vi "KoordListGUI.vi"() -> ()   [LabVIEW 2011]
uses:
  <vilib>/Utility/error.llb/whitespace.ctl
panel:
  in  "Detector":u16(ring) items=["scan", "pike"]
  in  "Positions":i32=12
  in  "Registerkarte":T1(tab)=enum."Size"
  in  "Save":bool
  in  "Load":bool
  in  "slide-center [m]":cluster{"X":dbl, "Y":dbl}={"X"=0.0106, "Y"=0.004}
  in  "slide-size [m]":cluster{"X":dbl, "Y":dbl}={"X"=0.02, "Y"=0.01}
  in  "step":cluster{"Stepx":dbl, "Stepy":dbl}={"Stepx"=0.0006, "Stepy"=0.0006} {"Stepy" format="%#_6p"; "Stepx" format="%#_6p"}
  out "Objective X":dbl=10.0
  in  "ReadSize":bool
  out "y":i32=3
  out "x":i32=4
  in  "max":cluster{"maxX":dbl, "maxY":dbl}={"maxX"=0.011708333333333331, "maxY"=0.0028645833333333336} {"maxY" format="%#_6p"; "maxX" format="%#_6p"}
  in  "min":cluster{"MinX":dbl, "MinY":dbl}={"MinX"=0.0044166666666666625, "MinY"=-0.0031249999999999993} {"MinY" format="%#_6p"; "MinX" format="%#_6p"}
  out "Image":T2(plugin-control)
  in  "create list":bool
  out "Mouse position":cluster{"x":dbl, "y":dbl}={"x"=1.9429894176211716e-14, "y"=99.99999999999996} {"y" format="%#_6p"; "x" format="%#_6p"}
  in  "List":i32(listbox)=-1
  out "experimet":string="steve7"
  in  "Cancel":bool
  in  "Run":bool
  in  "State":T3(ring)=enum."close"
  out "Next is":i32
  out "Numerisch":dbl=0.00474167
  out "String":string="stage.y.set"
  out "stage notification":string=" 0.011600 ,0.0000"
  in  "End":bool
  # "Coordinates"
  # "Till-stage: 0.01248/0.01235\nPrior: 0,05703/0,03722\nAsi is 0.006/0"
  # "default size 0.050/0.025"
  # "of last image \ndone with this\ndetector"
  # "(Image center!)"
  # "Debug"
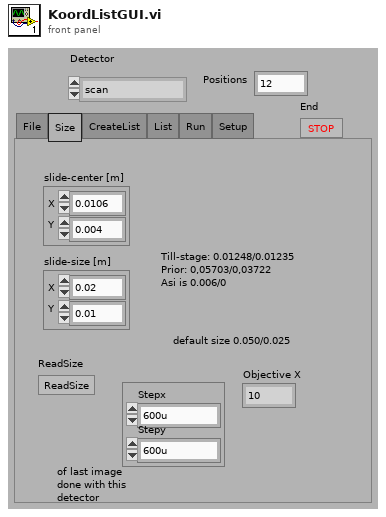
[diagram p1: front panel]
types:
  T1 = enum32{"File", "Size", "CreateList", "List", "Run", "Setup"}
  T2 = typedef "IMAQ Image.ctl" = refnum<image>
  T3 = enum16{"idle", "start", "move", "image", "stop", "close"}
  T4 = enum16{"None/#Datasets", "Clear", "TagValueOf#", "AddValues", "ReadValue", "ChangeValue", "Get all"}
  T5 = typedef "Image Type" = u32
  T6 = typedef "whitespace.ctl" = u16
  T7 = cluster{"Global Rectangle":i32[], "Contours":cluster{"Contour Type":u32, "ROI Type":u32, "Points":i32[]}[]}
  T8 = typedef "IMAQ Rectangle" = cluster{"Left":i32, "Top":i32, "Right":i32, "Bottom":i32, "Rotation":dbl}
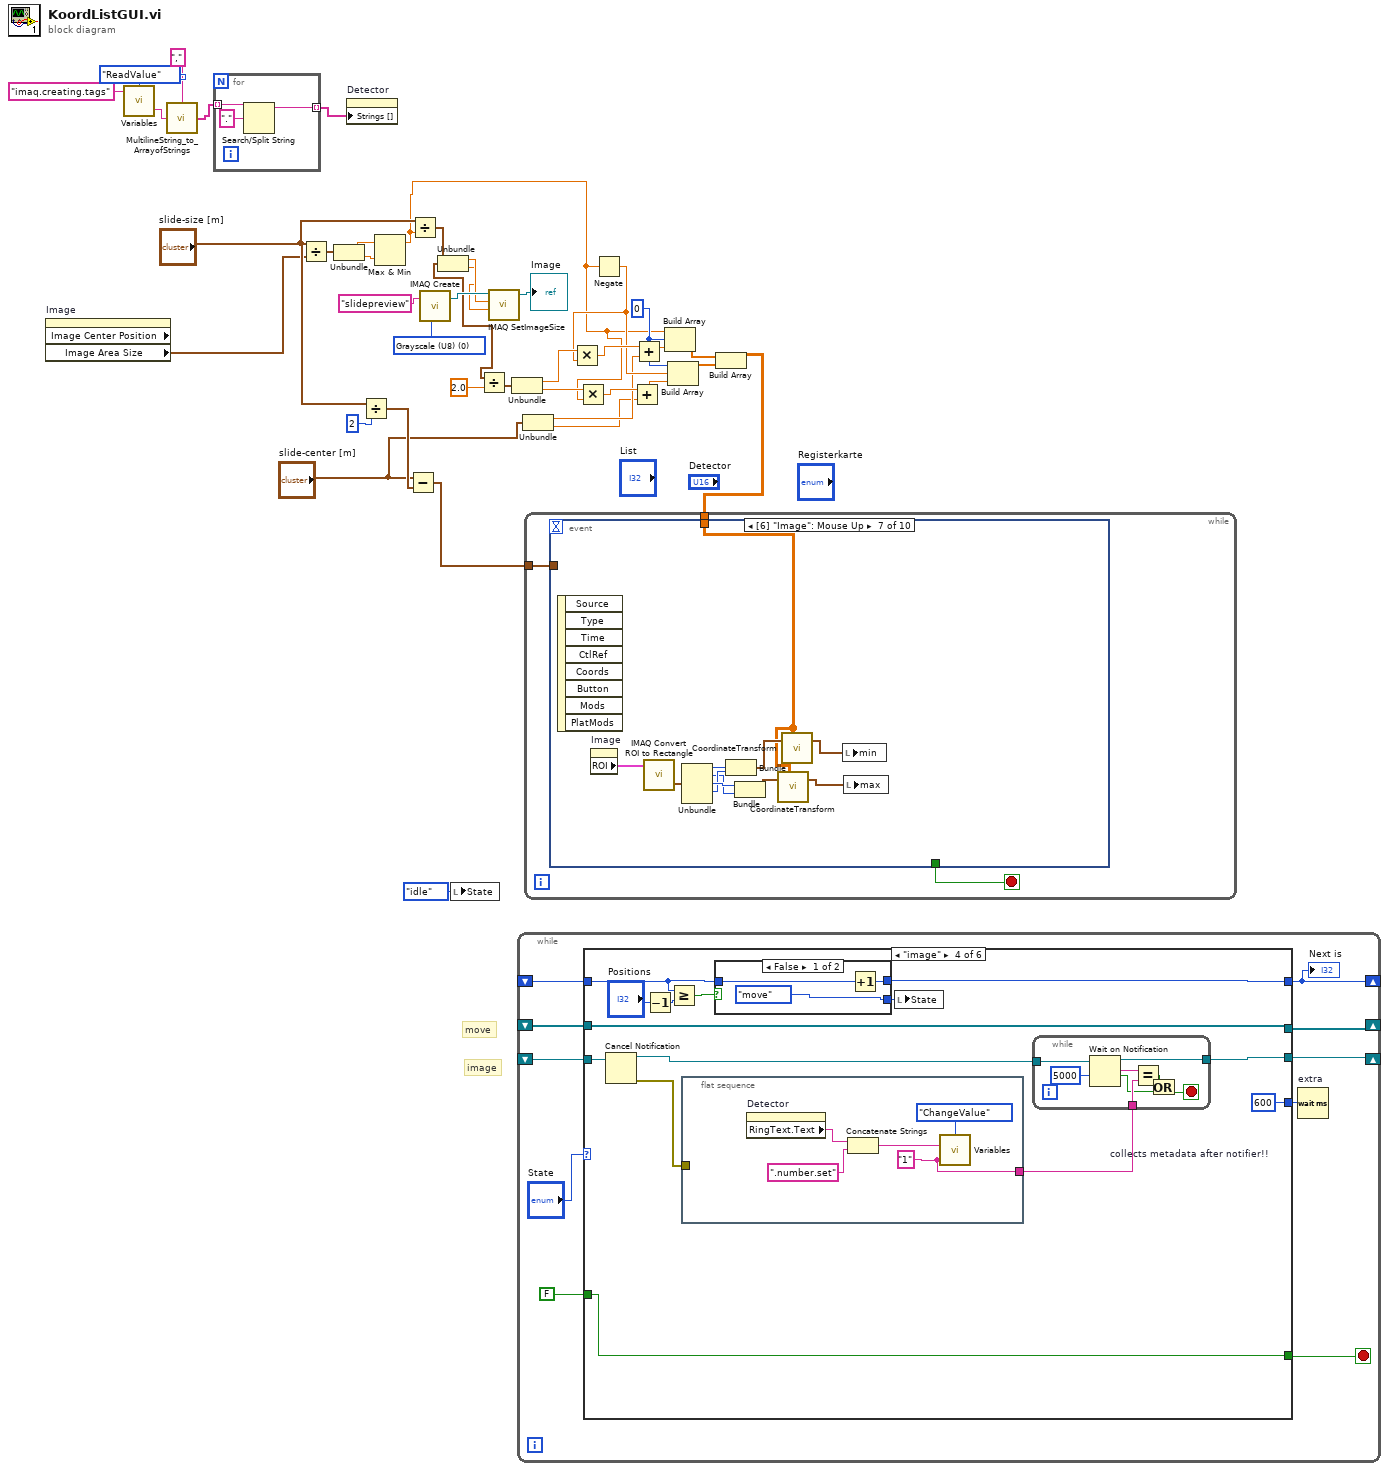
[diagram p0: block diagram]
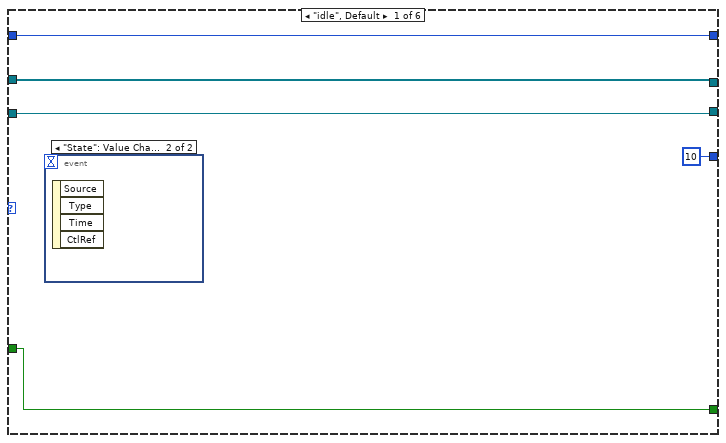
[diagram p2: hidden frame]
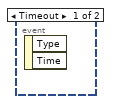
[diagram p3: hidden frame]
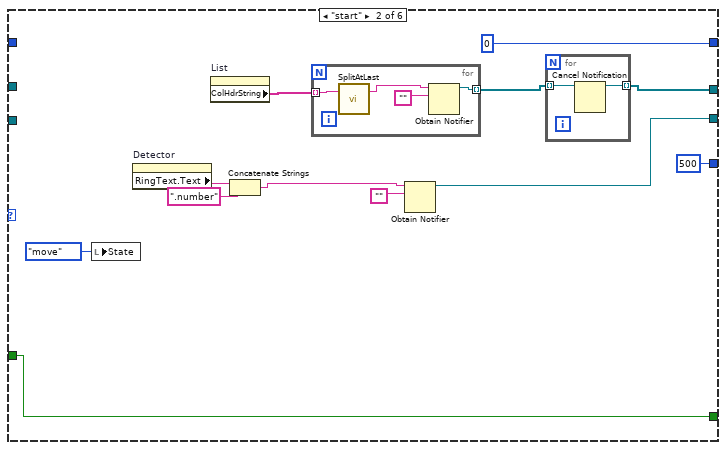
[diagram p4: hidden frame]
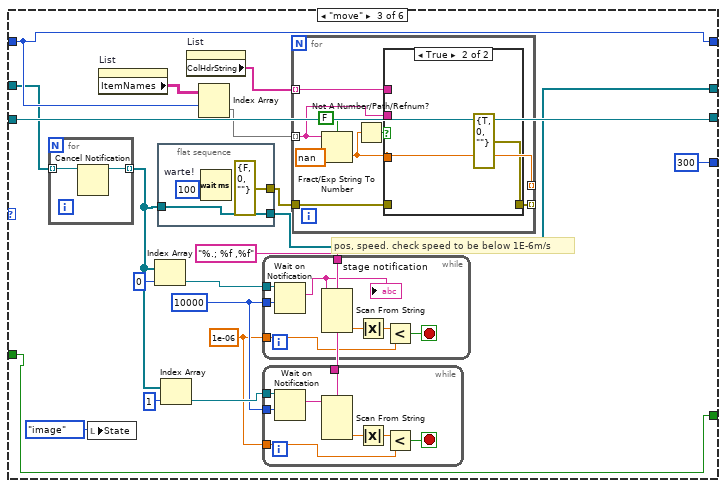
[diagram p5: hidden frame]
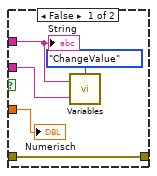
[diagram p6: hidden frame]
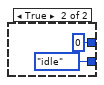
[diagram p7: hidden frame]
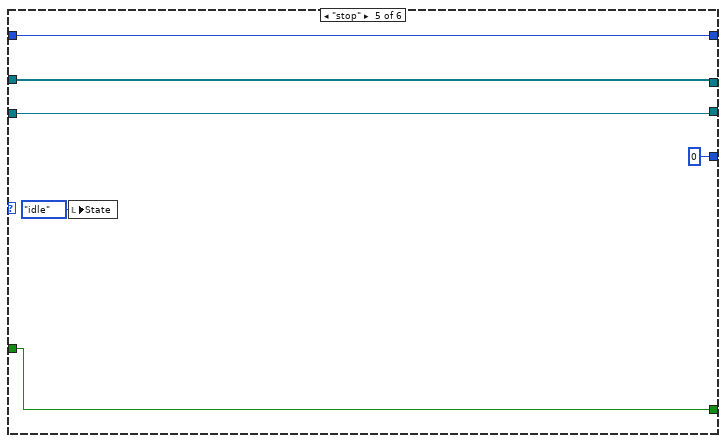
[diagram p8: hidden frame]
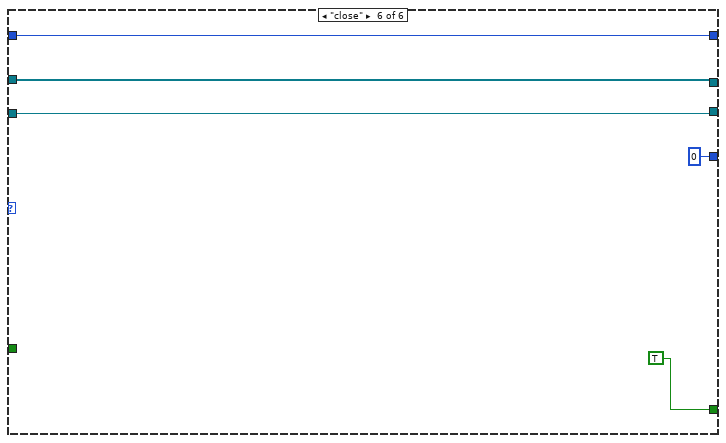
[diagram p9: hidden frame]
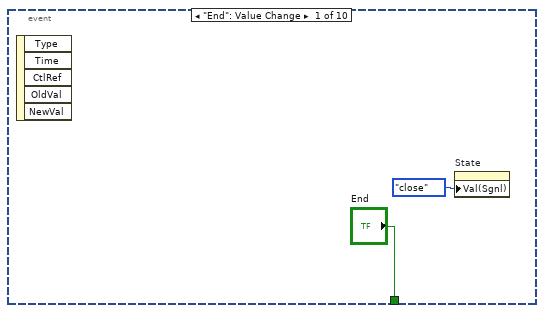
[diagram p10: hidden frame]
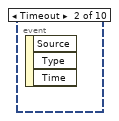
[diagram p11: hidden frame]
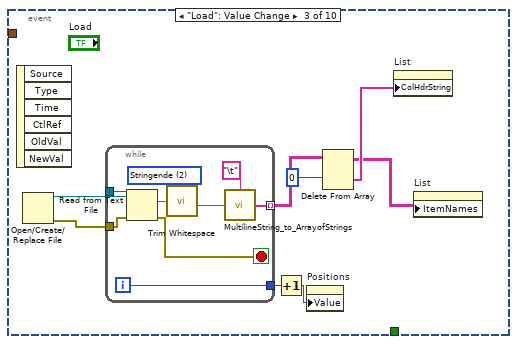
[diagram p12: hidden frame]
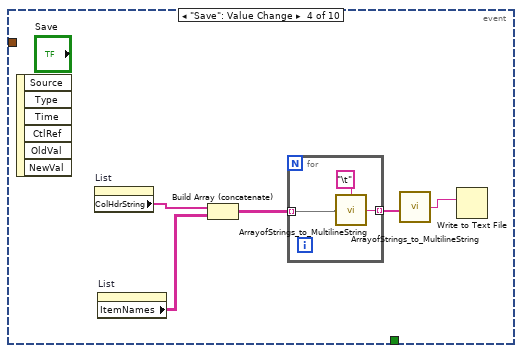
[diagram p13: hidden frame]
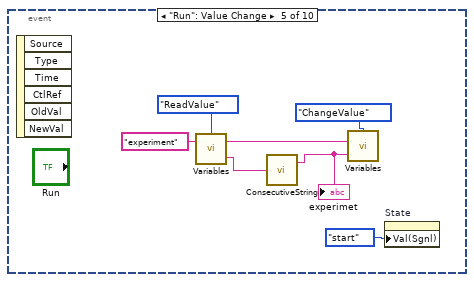
[diagram p14: hidden frame]
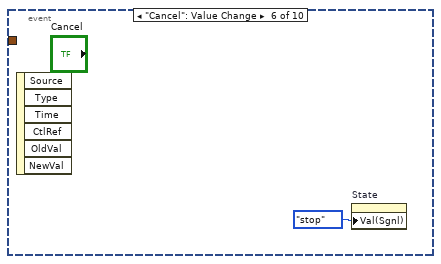
[diagram p15: hidden frame]
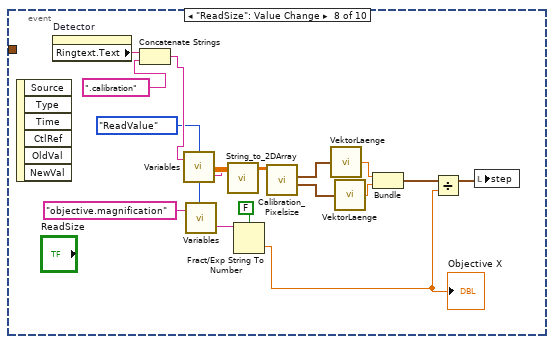
[diagram p16: hidden frame]
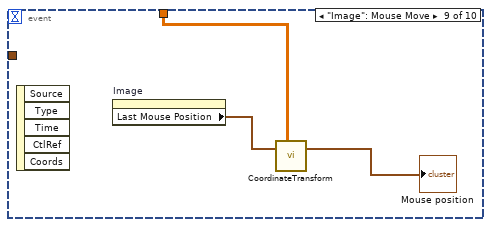
[diagram p17: hidden frame]
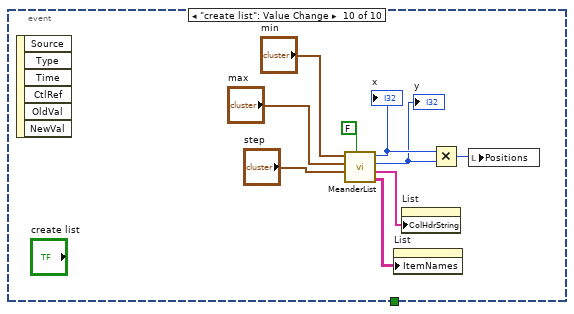
[diagram p18: hidden frame]
diagram:
  w23 = 0
  w38 = T5 0 items=["Grayscale (U8)", "Grayscale (I16)", "Grayscale (SGL)", "Complex (CSG)", "RGB (U32)", "HSL (U32)", "RGB (U64)"] ("Image Type")
  # "image"
  # "move"
  n1 = property on="Image" class="ImageControl" props=["Image Center Position", "Image Area Size"]() -> ("Image Area Size"=w21:cluster{"Width":u32, "Height":u32})  [unwired: 2 in, 3 out]
  n2 = call "Variables.vi"("Tag in"="imaq.creating.tags", "Command"=T4."ReadValue") -> ("value out"=w11:string)  [unwired: 1 in, 2 out]
  n3 = call "MultilineString_to_ArrayofStrings.vi"("String 1"=w11, "NewLineString"=",") -> ("String Array"=w9:string[])
  n4 = for {
    tunnel: w9 -> [w42] mode=indexing
    tunnel: [w41] -> w8 mode=indexing
    n5 = Search/Split String(string=w42, search string/char (-)=".") -> (substring before match=w41:string)  [unwired: 1 in, 2 out]
  }
  n6 = Divide(x="slide-size [m]", y=w21) -> (x/y=w34:cluster{dbl, dbl})
  n7 = Unbundle(w34) -> (w33:dbl, w32:dbl)
  n8 = property on="Detector" class="Ring (strict)"("Strings []"=w8) -> ()  [unwired: 2 in, 2 out]
  n9 = Divide(x="slide-size [m]", y=2) -> (x/y=w28:cluster{"X":dbl, "Y":dbl})
  n10 = Max & Min(x=w33, y=w32) -> (max(x,y)=w14:dbl)  [unwired: 1 out]
  n11 = Subtract(x="slide-center [m]", y=w28) -> (x-y=w27:cluster{"X":dbl, "Y":dbl})
  n12 = Divide(x="slide-size [m]", y=w14) -> (x/y=w18:cluster{"X":dbl, "Y":dbl})
  n13 = call "IMAQ Create"("Image Name"="slidepreview", "Image Type"=w38) -> ("New Image"=w37:T2)  [unwired: 2 in, 2 out]
  n14 = Unbundle(w18) -> ("X"=w36:dbl, "Y"=w35:dbl)
  n15 = local write "State"(T3."idle" ("State")) -> ()
  n16 = Divide(x=w18, y=2.0) -> (x/y=w17:cluster{"X":dbl, "Y":dbl})
  n17 = call "IMAQ SetImageSize"("Y Resolution"=w35, "X Resolution"=w36, "Image"=w37) -> ("Image Out"=→"Image":T2)  [unwired: 1 in, 2 out]
  n18 = Unbundle(w17) -> ("X"=w20:dbl, "Y"=w19:dbl)
  n19 = while {
    shift-right: [w51] -> _
    shift-left: _ -> [w52]
    shift-right: [w50] -> _
    shift-left: _ -> [w49]
    shift-right: [w44] -> _
    shift-left: _ -> [w48]
    stop <- w47 stop-if-true
    n20 = case shown="\"image\"" "State" {
      tunnel: w52 -> [w57 _ w82 w143 w166 w171]
      tunnel: [w57 w61 w81 w143 w166 w171] -> w51
      tunnel: [w56 w67 w94 w142 w165 w170] -> w50
      tunnel: w49 -> [w56 _ w94 w132 w165 w170]
      tunnel: w48 -> [w55 _ w89 w137 w167 w172]
      tunnel: [w55 0 w89 w136 w167 w172] -> w44
      tunnel: [w54 w65 w80 w140 w164 TRUE] -> w47
      tunnel: FALSE -> [w54 w65 w80 w140 w164 _]
      tunnel: [u32 10 ("Zu wartende ms") u32 500 ("Zu wartende ms") u32 300 ("Zu wartende ms") w134 u32 0 ("Zu wartende ms") u32 0 ("Zu wartende ms")] -> w43
      frame "idle", Default {
        n21 = event shown="[1] \"State\": Value Change" {
          selector: _ -> [_ _]
          dyn-events: _ -> [_ _]
          timeout: _ -> [_ _]
          event Timeout {
            n22 = event-data() -> ()  [unwired: 3 out]
          }
          event "State": Value Change {
            n23 = event-data() -> ()  [unwired: 5 out]
          }
        }
      }
      frame "start" {
        n24 = local write "State"(T3."move" ("State")) -> ()
        n25 = property on="Detector" class="Ring (strict)"() -> ("RingText.Text"=w60:string)  [unwired: 2 in, 2 out]
        n26 = property on="List" class="MCListbox (strict)"() -> ("ColHdrString"=w69:string[])  [unwired: 2 in, 2 out]
        n27 = Concatenate Strings(w60, ".number" ("string")) -> (w58:string)
        n28 = for {
          tunnel: w69 -> [w73] mode=indexing
          tunnel: [w74] -> w62 mode=indexing
          n29 = call "SplitAtLast.vi"("In-String"=w73) -> ("Front (default)"=w72:string)  [unwired: 1 in, 1 out]
          n30 = Obtain Notifier(name (unnamed)=w72, notification data type="") -> (notifier out=w74:refnum<notifier>)  [unwired: 2 in, 2 out]
        }
        n31 = Obtain Notifier(name (unnamed)=w58, notification data type="") -> (notifier out=w67:refnum<notifier>)  [unwired: 2 in, 2 out]
        n32 = for {
          tunnel: w62 -> [w71] mode=indexing
          tunnel: [w70] -> w61 mode=indexing
          n33 = Cancel Notification(0:w71) -> (8:w70:refnum<notifier>)  [unwired: 1 in, 2 out]
        }
      }
      frame "move" {
        w77 = 1e-06 ("y")
        w76 = "%.; %f ,%f" ("format string")
        w78 = 10000 ("Timeout in ms(-1)")
        # "pos, speed. check speed to be below 1E-6m/s"
        n34 = for {
          tunnel: w82 -> [w115] mode=indexing
          tunnel: [w114] -> w83 mode=indexing
          n35 = Cancel Notification(0:w115) -> (8:w114:refnum<notifier>)  [unwired: 1 in, 2 out]
        }
        n36 = local write "State"(T3."image" ("State")) -> ()
        n37 = property on="List" class="MCListbox (strict)"() -> ("ItemNames"=w93:string[][])  [unwired: 2 in, 2 out]
        n38 = Index Array(array=w83, index=0 ("Index")) -> (element=w85:refnum<notifier>)
        n39 = flat-sequence {
          tunnel: [errorcluster {"status"=FALSE, "code"=0, "source"=""} ("Fehler (Eingang, kein Fehler)")] -> w90
          tunnel: w83 -> [w111]
          tunnel: [w111] -> w81
          frame #0 {
            w112 = u32 100  # warte!
            n40 = Wait (ms)(milliseconds to wait=w112) -> ()  [unwired: 1 out]
          }
        }
        n41 = Index Array(array=w83, index=1 ("Index")) -> (element=w79:refnum<notifier>)
        n42 = property on="List" class="MCListbox (strict)"() -> ("ColHdrString"=w91:string[])  [unwired: 2 in, 2 out]
        n43 = Index Array(array=w93, index (row)=w89) -> (element=w92:string[])  [unwired: 1 in]
        n44 = while {
          tunnel: w85 -> [w110]
          tunnel: w78 -> [w109]
          tunnel: w77 -> [w104]
          tunnel: w76 -> [w103]
          stop <- w105 stop-if-true
          n45 = Wait on Notification(notifier=w110, timeout in ms (-1)=w109) -> (notification=w108:string)  [unwired: 1 in, 4 out]
          "stage notification" <- w108
          n46 = Scan From String(format string=w103, input string=w108) -> (output 2=w107:dbl)  [unwired: 5 in, 3 out]
          n47 = Absolute Value(x=w107) -> (abs(x)=w106:dbl)
          n48 = Less?(x=w106, y=w104) -> (x < y?=w105:bool)
        }
        n49 = while {
          tunnel: w79 -> [w102]
          tunnel: w78 -> [w101]
          tunnel: w77 -> [w96]
          tunnel: w76 -> [w95]
          stop <- w97 stop-if-true
          n50 = Wait on Notification(notifier=w102, timeout in ms (-1)=w101) -> (notification=w100:string)  [unwired: 1 in, 4 out]
          n51 = Scan From String(format string=w95, input string=w100) -> (output 2=w99:dbl)  [unwired: 5 in, 3 out]
          n52 = Absolute Value(x=w99) -> (abs(x)=w98:dbl)
          n53 = Less?(x=w98, y=w96) -> (x < y?=w97:bool)
        }
        n54 = for {
          tunnel: w91 -> [w120] mode=indexing
          tunnel: w92 -> [w119] mode=indexing
          tunnel: [w116] -> _ mode=indexing
          tunnel: w90 -> [w118]
          tunnel: [w117] -> _ mode=indexing
          n55 = Fract/Exp String To Number(use system decimal point (T)=FALSE ("Systemdezimalzeichen verwenden (T)"), string=w119, default (0 dbl)=nan ("Standard (0 DBL)")) -> (number=w116:dbl)  [unwired: 2 out]
          n56 = Not A Number/Path/Refnum?(number/path/refnum=w116) -> (NaN/Path/Refnum?=w121:bool)
          n57 = case shown="True" w121 {
            tunnel: w116 -> [w128 _]
            tunnel: w120 -> [w126 _]
            tunnel: w119 -> [w127 _]
            tunnel: w118 -> [w124 _]
            tunnel: [w124 errorcluster {"status"=TRUE, "code"=0, "source"=""} ("Fehler (Eingang, kein Fehler)")] -> w117
            frame False {
              n58 = call "Variables.vi"("value"=w127, "Tag in"=w126, "Command"=T4."ChangeValue") -> ()  [unwired: 3 out]
              "String" <- w126
              "Numerisch" <- w128
            }
            frame True {
            }
          }
        }
      }
      frame "image" {
        w134 = u32 600  # collects metadata after notifier!!
        n59 = Cancel Notification(0:w132) -> (8:w131:refnum<notifier>, 11:w130:errorcluster)  [unwired: 1 in, 1 out]
        n60 = Decrement(x="Positions") -> (x-1=w133:i32)
        n61 = Greater Or Equal?(x=w137, y=w133) -> (x >= y?=w138:bool)
        n62 = flat-sequence {
          tunnel: [w144] -> w141
          tunnel: w130 -> [_]
          frame #0 {
            w144 = "1" ("value")
            n63 = property on="Detector" class="Ring (strict)"() -> ("RingText.Text"=w147:string)  [unwired: 2 in, 2 out]
            n64 = Concatenate Strings(w147, ".number.set" ("execute")) -> (w145:string)
            n65 = call "Variables.vi"("value"=w144, "Tag in"=w145, "Command"=T4."ChangeValue") -> ()  [unwired: 3 out]
          }
        }
        n66 = case shown="False" w138 {
          tunnel: w137 -> [w151 _]
          tunnel: [w150 0] -> w136
          tunnel: [T3."move" ("State") T3."idle" ("State")] -> w135
          frame False {
            n67 = Increment(x=w151) -> (x+1=w150:i32)
          }
          frame True {
          }
        }
        n68 = local write "State"(w135) -> ()
        n69 = while {
          tunnel: w131 -> [w161]
          tunnel: [w160] -> w142
          tunnel: w141 -> [w157]
          stop <- w155 stop-if-true
          n70 = Wait on Notification(notifier=w161, timeout in ms (-1)=5000 ("Timeout in ms(-1)")) -> (notifier out=w160:refnum<notifier>, notification=w158:string, timed out?=w154:bool)  [unwired: 1 in, 2 out]
          n71 = Equal?(x=w158, y=w157) -> (x = y?=w156:bool)
          n72 = Or(x=w156, y=w154) -> (x .or. y?=w155:bool)
        }
      }
      frame "stop" {
        n73 = local write "State"(T3."idle" ("State")) -> ()
      }
      frame "close" {
      }
    }
    "Next is" <- w44
    n74 = Wait (ms) "extra"(milliseconds to wait=w43) -> ()  [unwired: 1 out]
  }
  n75 = Unbundle("slide-center [m]") -> ("X"=w3:dbl, "Y"=w2:dbl)
  n76 = Multiply(x=w19, y=w14) -> (x*y=w4:dbl)
  n77 = Negate(x=w14) -> (-x=w15:dbl)
  n78 = Multiply(x=w20, y=w15) -> (x*y=w16:dbl)
  n79 = Add(x=w4, y=w2) -> (x+y=w5:dbl)
  n80 = Add(x=w16, y=w3) -> (x+y=w6:dbl)
  n81 = Build Array(w14, w23, w6) -> (w25:dbl[])
  n82 = Build Array(w23, w15, w5) -> (w24:dbl[])
  n83 = Build Array(w25, w24) -> (w1:dbl[][])
  n84 = while {
    tunnel: w27 -> [w174]
    tunnel: w1 -> [w173]
    stop <- w175 stop-if-true
    n85 = event shown="[6] \"Image\": Mouse Up" {
      selector: _ -> [_ _ _ _ _ _ _ _ _ _]
      dyn-events: _ -> [_ _ _ _ _ _ _ _ _ _]
      timeout: _ -> [_ _ _ _ _ _ _ _ _ _]
      tunnel: ["End" _ _ _ _ _ _ _ _ _] -> w175
      tunnel: w174 -> [_ _ _ _ _ _ _ _ _ _]
      tunnel: w173 -> [_ _ _ _ _ _ w213 _ w238 _]
      event "End": Value Change {
        n86 = event-data() -> ()  [unwired: 6 out]
        n87 = property on="State" class="Enum (strict)"("Val(Sgnl)"=T3."close" ("Wert (signalisierend)")) -> ()  [unwired: 2 in, 2 out]
      }
      event Timeout {
        n88 = event-data() -> ()  [unwired: 4 out]
      }
      event "Load": Value Change {
        n89 = event-data() -> ()  [unwired: 7 out]
        n90 = Open/Create/Replace File() -> (refnum out=w185:refnum<file>, error out=w184:errorcluster)  [unwired: 1 in, 6 out]
        n91 = while {
          tunnel: w185 -> [w194]
          tunnel: w184 -> [w192]
          tunnel: [w189] -> w180 mode=indexing
          tunnel: [w186] -> w179
          i -> [w186]
          stop <- w193 stop-if-true
          w187 = T6 2 items=["beide", "Stringanfang", "Stringende"] ("location (both)")
          n92 = Read from Text File(file (use dialog)=w194, error in=w192) -> (text=w190:string, error out=w193:errorcluster)  [unwired: 4 out]
          n93 = call <vilib>:"Trim Whitespace.vi"("string"=w190, "location (both)"=w187) -> ("trimmed string"=w188:string)
          n94 = call "MultilineString_to_ArrayofStrings.vi"("String 1"=w188, "NewLineString"="\t") -> ("String Array"=w189:string[])
        }
        n95 = Increment(x=w179) -> (x+1=w178:i32)
        n96 = property on="Positions" class="DigNum (strict)"("Value"=w178) -> ()  [unwired: 2 in, 2 out]
        n97 = Delete From Array(array=w180, index (row)=0 ("Index (Zeile)")) -> (deleted portion=w182:string[], array with subset deleted=w181:string[][])  [unwired: 2 in]
        n98 = property on="List" class="MCListbox (strict)"("ColHdrString"=w182) -> ()  [unwired: 2 in, 2 out]
        n99 = property on="List" class="MCListbox (strict)"("ItemNames"=w181) -> ()  [unwired: 2 in, 2 out]
      }
      event "Save": Value Change {
        n100 = event-data() -> ()  [unwired: 7 out]
        n101 = property on="List" class="MCListbox (strict)"() -> ("ColHdrString"=w199:string[])  [unwired: 2 in, 2 out]
        n102 = property on="List" class="MCListbox (strict)"() -> ("ItemNames"=w198:string[][])  [unwired: 2 in, 2 out]
        n103 = Build Array (concatenate)(w199, w198) -> (w197:string[][])
        n104 = for {
          tunnel: w197 -> [w202] mode=indexing
          tunnel: [w200] -> w196 mode=indexing
          n105 = call "ArrayofStrings_to_MultilineString.vi"("String Array"=w202, "NewLineString"="\t") -> ("String 1"=w200:string)
        }
        n106 = call "ArrayofStrings_to_MultilineString.vi"("String Array"=w196) -> ("String 1"=w195:string)  [unwired: 1 in]
        n107 = Write to Text File(text=w195) -> ()  [unwired: 1 in, 5 out]
      }
      event "Run": Value Change {
        n108 = event-data() -> ()  [unwired: 7 out]
        n109 = call "Variables.vi"("Tag in"="experiment", "Command"=T4."ReadValue") -> ("value out"=w206:string, "Tag out"=w204:string)  [unwired: 1 in, 1 out]
        n110 = call "ConsecutiveString.vi"("String"=w206) -> ("Consecutive String"=w205:string)  [unwired: 1 out]
        "experimet" <- w205
        n111 = call "Variables.vi"("value"=w205, "Tag in"=w204, "Command"=T4."ChangeValue") -> ()  [unwired: 3 out]
        n112 = property on="State" class="Enum (strict)"("Val(Sgnl)"=T3."start" ("Wert (signalisierend)")) -> ()  [unwired: 2 in, 2 out]
      }
      event "Cancel": Value Change {
        n113 = event-data() -> ()  [unwired: 7 out]
        n114 = property on="State" class="Enum (strict)"("Val(Sgnl)"=T3."stop" ("Wert (signalisierend)")) -> ()  [unwired: 2 in, 2 out]
      }
      event "Image": Mouse Up {
        n115 = event-data() -> ()  [unwired: 9 out]
        n116 = property on="Image" class="ImageControl"() -> ("ROI"=w221:T7)  [unwired: 2 in, 2 out]
        n117 = call "IMAQ Convert ROI to Rectangle"("ROI Descriptor"=w221) -> ("Rectangle"=w220:T8)  [unwired: 1 in, 8 out]
        n118 = Unbundle(w220) -> ("Left"=w219:i32, "Top"=w211:i32, "Right"=w218:i32, "Bottom"=w212:i32)  [unwired: 1 out]
        n119 = Bundle("Left"=w219, "Bottom"=w212) -> (w217:cluster{"Left":i32, "Bottom":i32})  [unwired: 1 out]
        n120 = Bundle("Right"=w218, "Top"=w211) -> (w215:cluster{"Right":i32, "Top":i32})  [unwired: 1 out]
        n121 = call "CoordinateTransform.vi"("input coordiantes"=w215, "Conversion Matrix"=w213) -> ("output coordiantes"=w214:cluster{"x":dbl, "y":dbl})  [unwired: 2 in, 1 out]
        n122 = call "CoordinateTransform.vi"("input coordiantes"=w217, "Conversion Matrix"=w213) -> ("output coordiantes"=w216:cluster{"x":dbl, "y":dbl})  [unwired: 2 in, 1 out]
        n123 = local write "min"(w216) -> ()
        n124 = local write "max"(w214) -> ()
      }
      event "ReadSize": Value Change {
        w226 = T4."ReadValue" ("Command")
        n125 = event-data() -> ()  [unwired: 7 out]
        n126 = property on="Detector" class="Ring (strict)"() -> ("Ringtext.Text"=w229:string)  [unwired: 2 in, 2 out]
        n127 = Concatenate Strings(w229, ".calibration" ("Search")) -> (w227:string)
        n128 = call "Variables.vi"("Tag in"=w227, "Command"=w226) -> ("value out"=w236:string)  [unwired: 1 in, 2 out]
        n129 = call "Variables.vi"("Tag in"="objective.magnification", "Command"=w226) -> ("value out"=w224:string)  [unwired: 1 in, 2 out]
        n130 = call "String_to_2DArray.vi"("String"=w236) -> ("Array"=w237:dbl[][])  [unwired: 3 in, 1 out]
        n131 = Fract/Exp String To Number(use system decimal point (T)=FALSE, string=w224) -> (number=w222:dbl)  [unwired: 2 in, 1 out]
        "Objective X" <- w222
        n132 = call "Calibration_Pixelsize.vi"("CalibrationCoordinates: x,x'y,y'..."=w237) -> ("slow"=w234:cluster{"x'":dbl, "y'":dbl}, "Fast"=w235:cluster{"x'":dbl, "y'":dbl})  [unwired: 9 out]
        n133 = call "VektorLaenge.vi"("Vektor"=w235) -> ("Vektorlänge"=w233:dbl)
        n134 = call "VektorLaenge.vi"("Vektor"=w234) -> ("Vektorlänge"=w232:dbl)
        n135 = Bundle("Vektorlänge"=w233, "Vektorlänge"=w232) -> (w231:cluster{"Vektorlänge":dbl, "Vektorlänge":dbl})  [unwired: 1 in]
        n136 = Divide(x=w231, y=w222) -> (x/y=w230:cluster{"Vektorlänge":dbl, "Vektorlänge":dbl})
        n137 = local write "step"(w230) -> ()
      }
      event "Image": Mouse Move {
        n138 = event-data() -> ()  [unwired: 6 out]
        n139 = property on="Image" class="ImageControl"() -> ("Last Mouse Position"=w239:cluster{"X":i32, "Y":i32})  [unwired: 2 in, 2 out]
        n140 = call "CoordinateTransform.vi"("input coordiantes"=w239, "Conversion Matrix"=w238) -> ("output coordiantes"=→"Mouse position":cluster{"x":dbl, "y":dbl})  [unwired: 2 in, 1 out]
      }
      event "create list": Value Change {
        n141 = event-data() -> ()  [unwired: 7 out]
        n142 = call "MeanderList.vi"("single side"=FALSE ("Mäander"), "step"="step", "max"="max", "min"="min") -> ("Positions"=w244:string[][], "Axis"=w245:string[], "y"=w242:i32, "x"=w243:i32)  [unwired: 4 out]
        "x" <- w243
        "y" <- w242
        n143 = property on="List" class="MCListbox (strict)"("ItemNames"=w244) -> ()  [unwired: 2 in, 2 out]
        n144 = property on="List" class="MCListbox (strict)"("ColHdrString"=w245) -> ()  [unwired: 2 in, 2 out]
        n145 = Multiply(x=w243, y=w242) -> (x*y=w241:i32)
        n146 = local write "Positions"(w241) -> ()
      }
    }
  }
